vi "GetSraight EdgeResultNameUsed Edges.vi"(8 "Number of Matches Requested":i32, 9 "string":string, 10 "String":string, 11 "element":refnum<vi>) -> (3 "Array":string[](array[string]))   [LabVIEW 2015]
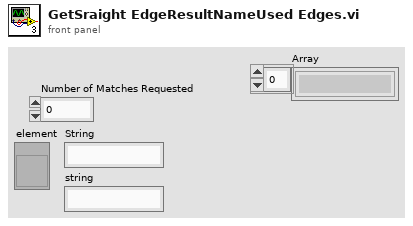
[diagram p1: front panel]
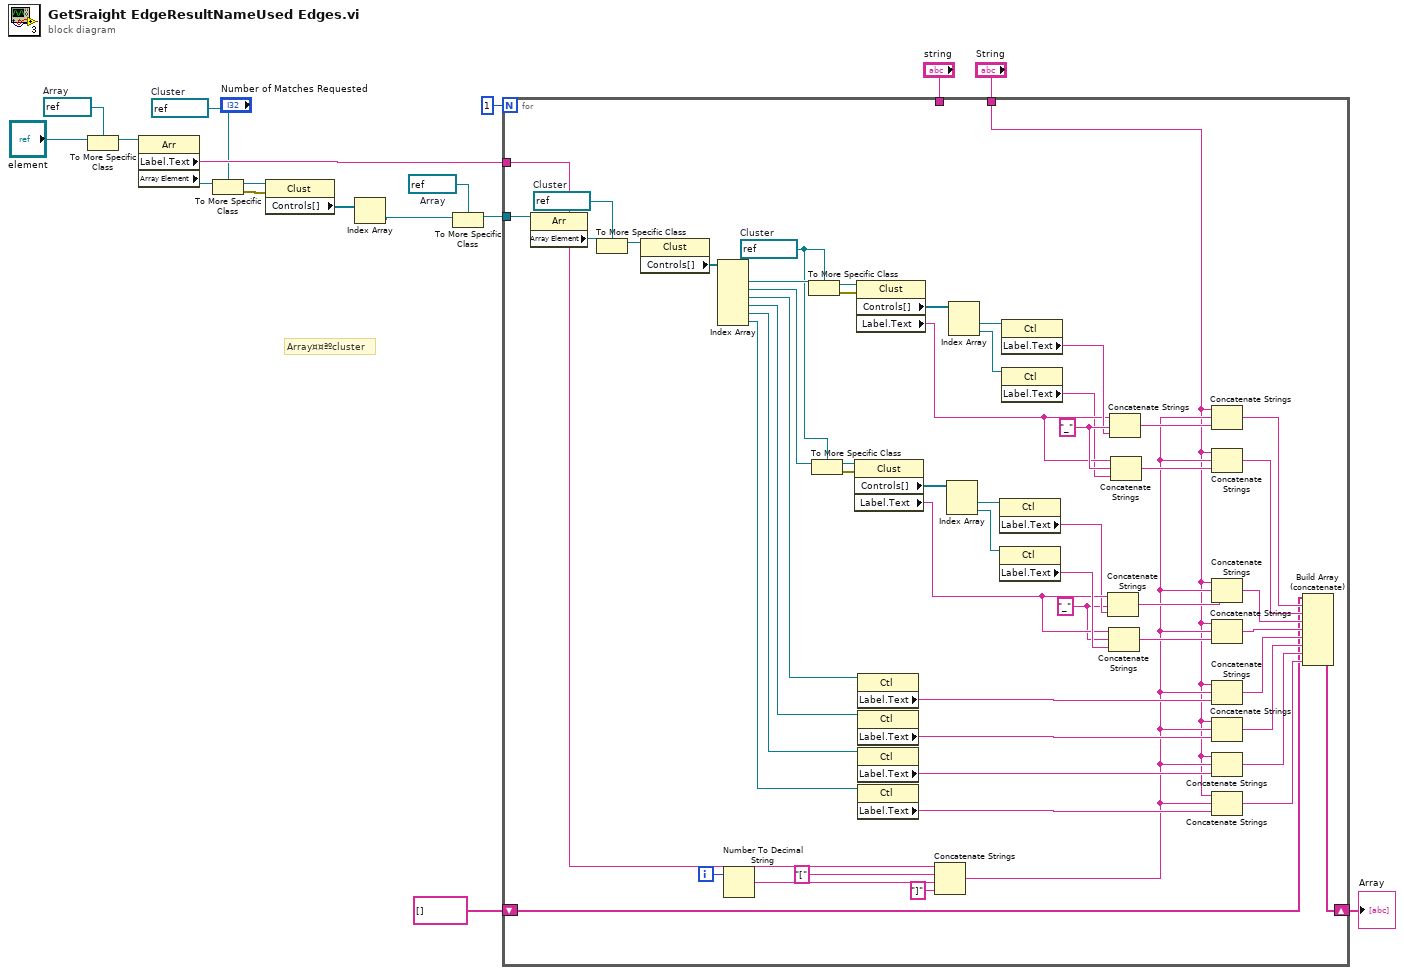
[diagram p0: block diagram]
diagram:
  w15 = refnum<vi> refnum  # Array
  w7 = refnum<vi> refnum  # Cluster
  w9 = refnum<vi> refnum  # Array
  # "Array¤¤ªºcluster"
  n1 = To More Specific Class(target class=w9, reference="element") -> (specific class reference=w8:refnum<vi>)  [unwired: 1 in, 1 out]
  n2 = property class="Arr"(reference=w8) -> ("Label.Text"=w11:string, "Array Element"=w6:refnum<vi>)  [unwired: 1 in, 2 out]
  n3 = To More Specific Class(target class=w7, reference=w6) -> (specific class reference=w12:refnum<vi>, error out=w13:errorcluster)  [unwired: 1 in]
  n4 = property class="Clust"(reference=w12, error in=w13) -> ("Controls[]"=w14:refnum<vi>[])  [unwired: 2 out]
  n5 = Index Array(array=w14) -> (element=w16:refnum<vi>)  [unwired: 1 in]
  n6 = To More Specific Class(target class=w15, reference=w16) -> (specific class reference=w17:refnum<vi>)  [unwired: 1 in, 1 out]
  n7 = for {
    N: 1 -> [_]
    tunnel: w11 -> [w71]
    tunnel: w17 -> [w67]
    tunnel: "String" -> [w18]
    tunnel: "string" -> [_]
    shift-right: [w19] -> w2
    shift-left: string[] [] -> [w20]
    i -> [w72]
    w49 = "_"
    w56 = "_"
    w42 = refnum<vi> refnum  # Cluster
    w62 = refnum<vi> refnum  # Cluster
    n8 = property class="Arr"(reference=w67) -> ("Array Element"=w66:refnum<vi>)  [unwired: 1 in, 2 out]
    n9 = To More Specific Class(target class=w62, reference=w66) -> (specific class reference=w65:refnum<vi>)  [unwired: 1 in, 1 out]
    n10 = property class="Clust"(reference=w65) -> ("Controls[]"=w64:refnum<vi>[])  [unwired: 1 in, 2 out]
    n11 = Index Array(array=w64) -> (element #1=w63:refnum<vi>, element #2=w43:refnum<vi>, element #3=w41:refnum<vi>, element #4=w40:refnum<vi>, element #5=w39:refnum<vi>, element #6=w38:refnum<vi>)  [unwired: 6 in]
    n12 = Number To Decimal String(number=w72) -> (decimal integer string=w69:string)  [unwired: 1 in]
    n13 = To More Specific Class(target class=w42, reference=w63) -> (specific class reference=w61:refnum<vi>, error out=w60:errorcluster)  [unwired: 1 in]
    n14 = To More Specific Class(target class=w42, reference=w43) -> (specific class reference=w44:refnum<vi>, error out=w45:errorcluster)  [unwired: 1 in]
    n15 = property class="Clust"(reference=w44, error in=w45) -> ("Controls[]"=w46:refnum<vi>[], "Label.Text"=w51:string)  [unwired: 2 out]
    n16 = property class="Clust"(reference=w61, error in=w60) -> ("Controls[]"=w59:refnum<vi>[], "Label.Text"=w54:string)  [unwired: 2 out]
    n17 = property class="Ctl"(reference=w41) -> ("Label.Text"=w33:string)  [unwired: 1 in, 2 out]
    n18 = property class="Ctl"(reference=w40) -> ("Label.Text"=w32:string)  [unwired: 1 in, 2 out]
    n19 = property class="Ctl"(reference=w39) -> ("Label.Text"=w31:string)  [unwired: 1 in, 2 out]
    n20 = property class="Ctl"(reference=w38) -> ("Label.Text"=w30:string)  [unwired: 1 in, 2 out]
    n21 = Concatenate Strings(w71, "[" ("string"), w69, "]" ("string")) -> (w29:string)
    n22 = Index Array(array=w46) -> (element #1=w47:refnum<vi>, element #2=w48:refnum<vi>)  [unwired: 2 in]
    n23 = Index Array(array=w59) -> (element #1=w58:refnum<vi>, element #2=w57:refnum<vi>)  [unwired: 2 in]
    n24 = property class="Ctl"(reference=w47) -> ("Label.Text"=w50:string)  [unwired: 1 in, 2 out]
    n25 = property class="Ctl"(reference=w48) -> ("Label.Text"=w52:string)  [unwired: 1 in, 2 out]
    n26 = property class="Ctl"(reference=w58) -> ("Label.Text"=w55:string)  [unwired: 1 in, 2 out]
    n27 = property class="Ctl"(reference=w57) -> ("Label.Text"=w53:string)  [unwired: 1 in, 2 out]
    n28 = Concatenate Strings(w51, w49, w50) -> (w35:string)
    n29 = Concatenate Strings(w51, w49, w52) -> (w34:string)
    n30 = Concatenate Strings(w54, w56, w55) -> (w37:string)
    n31 = Concatenate Strings(w54, w56, w53) -> (w36:string)
    n32 = Concatenate Strings(w18, w29, w37) -> (w28:string)
    n33 = Concatenate Strings(w18, w29, w36) -> (w27:string)
    n34 = Concatenate Strings(w18, w29, w35) -> (w26:string)
    n35 = Concatenate Strings(w18, w29, w34) -> (w25:string)
    n36 = Concatenate Strings(w18, w29, w33) -> (w24:string)
    n37 = Concatenate Strings(w18, w29, w32) -> (w23:string)
    n38 = Concatenate Strings(w18, w29, w31) -> (w22:string)
    n39 = Concatenate Strings(w18, w29, w30) -> (w21:string)
    n40 = Build Array (concatenate)(w20, w28, w27, w26, w25, w24, w23, w22, w21) -> (w19:string[])
  }
  "Array" <- w2
